vi "exclude.set.vi"(8 "error in (no error)":errorcluster, 10 "exclude":set{refnum<class "filterTypes.lvclass">}(c389), 11 "exclude in":refnum<class "exclude.lvclass">) -> (0 "error out":errorcluster, 3 "exclude out":refnum<class "exclude.lvclass">)   [LabVIEW 2020, in "nominal types.lvlib" / "channelFilter.lvlib" / "exclude.lvclass"]
uses:
  exclude.lvclass
  exclude.lvclass/exclude.ctl
  filterTypes/filterTypes.lvclass
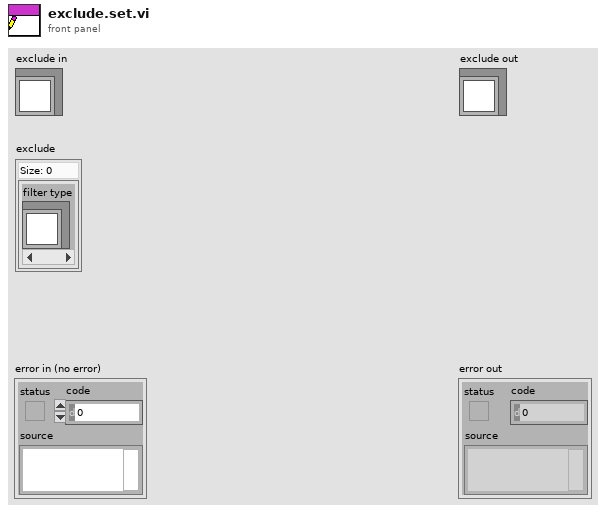
[diagram p1: front panel]
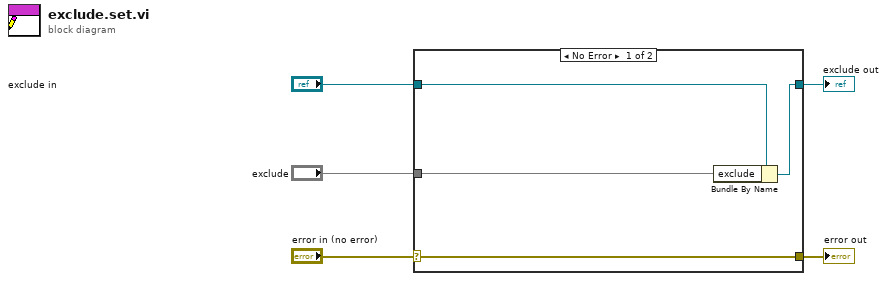
[diagram p0: block diagram]
diagram:
  n1 = case shown="No Error" "error in (no error)" {
    selector: "error in (no error)" -> [w9 w10]
    tunnel: [w9 w10] -> w4
    tunnel: [w7 w11] -> w2
    tunnel: "exclude in" -> [w8 w11]
    tunnel: "exclude" -> [w6 _]
    frame No Error {
      n2 = Bundle By Name(cluster=w8, "exclude"=w6) -> (w7:refnum<class "exclude.lvclass">)
    }
    frame Error {
    }
  }
  "error out" <- w4
  "exclude out" <- w2
